vi "WalkThroughExample.vi"() -> ()   [LabVIEW 2019]
uses:
  <vilib>/Rock Robotics/WPI/ThirdParty/JAS_Junk/TrajLib/LINEAR_SYSTEM.ctl
  <vilib>/Analysis/Matrix/Datatypes/RealMatrix.ctl
  <vilib>/Rock Robotics/WPI/ThirdParty/JAS_Junk/TrajLib/DCMOTOR.CTL
  <vilib>/Rock Robotics/WPI/ThirdParty/JAS_Junk/TrajLib/LINEAR_QUADRATIC_REGULATOR.ctl
  <vilib>/Rock Robotics/WPI/ThirdParty/JAS_Junk/TrajLib/KALMAN_FILTER.ctl
  <vilib>/Rock Robotics/WPI/ThirdParty/JAS_Junk/TrajLib/LINEAR_SYSTEM_LOOP.ctl
  <vilib>/Rock Robotics/WPI/ThirdParty/JAS_Junk/TrajLib/LINEAR_PLANT_INV_FF.ctl
  <vilib>/Rock Robotics/WPI/ThirdParty/JAS_Junk/TrajLib/FLYWHEEL_SIM.ctl
  <vilib>/Rock Robotics/WPI/ThirdParty/JAS_Junk/TrajLib/LINEAR_SYSTEM_SIM.ctl
  <vilib>/Rock Robotics/WPI/ThirdParty/JAS_Junk/TrajLib/DCMOTOR_TYPES_ENUM.ctl
  <vilib>/Rock Robotics/WPI/ThirdParty/JAS_Junk/TrajLib/MatBuilder_Create.vi
  <vilib>/Rock Robotics/WPI/ThirdParty/JAS_Junk/TrajLib/DCMotor_GetCIM.vi
  <vilib>/Rock Robotics/WPI/ThirdParty/JAS_Junk/TrajLib/DCMotor_GetAndymark9015.vi
  <vilib>/Rock Robotics/WPI/ThirdParty/JAS_Junk/TrajLib/DCMotor_GetAndymarkRs775_125.vi
  <vilib>/Rock Robotics/WPI/ThirdParty/JAS_Junk/TrajLib/DCMotor_GetBag.vi
  <vilib>/Rock Robotics/WPI/ThirdParty/JAS_Junk/TrajLib/DCMotor_GetBanebotsRs550.vi
  <vilib>/Rock Robotics/WPI/ThirdParty/JAS_Junk/TrajLib/DCMotor_GetBanebotsRs775.vi
  <vilib>/Rock Robotics/WPI/ThirdParty/JAS_Junk/TrajLib/DCMotor_GetFalcon500.vi
  <vilib>/Rock Robotics/WPI/ThirdParty/JAS_Junk/TrajLib/DCMotor_GetMiniCIM.vi
  <vilib>/Rock Robotics/WPI/ThirdParty/JAS_Junk/TrajLib/DCMotor_GetNEO.vi
  <vilib>/Rock Robotics/WPI/ThirdParty/JAS_Junk/TrajLib/DCMotor_GetNEO550.vi
  <vilib>/Rock Robotics/WPI/ThirdParty/JAS_Junk/TrajLib/DCMotor_GetRomiBuiltIn.vi
  <vilib>/Rock Robotics/WPI/ThirdParty/JAS_Junk/TrajLib/DCMotor_GetVex775Pro.vi
  <vilib>/Rock Robotics/WPI/ThirdParty/JAS_Junk/TrajLib/LinearSystem_New.vi
  <vilib>/Rock Robotics/WPI/ThirdParty/JAS_Junk/TrajLib/MatrixHelper_Zero.vi
  <vilib>/Rock Robotics/WPI/ThirdParty/JAS_Junk/TrajLib/MatBuilder_Fill.vi
  <vilib>/Rock Robotics/WPI/ThirdParty/JAS_Junk/TrajLib/Matrix_Ident.vi
  <vilib>/Rock Robotics/WPI/ThirdParty/JAS_Junk/TrajLib/DCMotor_New.vi
  <vilib>/Rock Robotics/WPI/ThirdParty/JAS_Junk/TrajLib/MatrixHelper_CoerceSize.vi
  <vilib>/Analysis/7linalg.llb/Create Special Matrix.vi
  <vilib>/Analysis/7linalg.llb/Create Special Real Matrix.vi
  <vilib>/Rock Robotics/WPI/ThirdParty/JAS_Junk/TrajLib/Trajectory_Library.lvlib
  <vilib>/ptbypt/NI_PtbyPt.lvlib
  <vilib>/Analysis/Matrix/NI_Matrix.lvlib
panel:
  in  "Tab Control":T1(tab)
  out "m_flywheelPlant":T2
  out "Shooter Motor":T4 {"Jr_KgM2" format="%13.5p"; "L_H" format="%13.5p"; "Kt_NMPerAmp" format="%13.5p"; "KvINV_RadPerSecPerVolt" format="%13.5p"; "R_Ohms" format="%13.5p"; "FreeSpeed_RadPerSec" format="%13.5p"; "FreeCurrent_Amps" format="%13.5p"; "StallCurrent_Amps" format="%13.5p"; "StallTorque_NM" format="%13.5p"; "nominalVoltage_Volts" format="%13.5p"}
  out "m_flywheelPlant_ALT":T2
  out "KalmanFilter":T5
  out "Kalman Creation Error":errorcluster
  out "LinearQuadraticRegulator":T6
  out "LQR Creation Error":bool
  out "Linear System Loop":T7
  out "LinSysLoop_Error":bool
  out "Battery Voltage":dbl format="%20.3f"
  out "CO Chart":cluster{dbl, "Voltage":dbl}(graph)
  in  "Shooter \nOn/Off":bool
  out "Encoder Speed\nRad/Sec":dbl(slide) scale=0.0..300.0
  out "Speed \nRad/Sec":dbl format="%16.1f"
  out "Cor Err":bool
  out "Kalman \nFiltered\nSpeed":dbl format="%16.1f"
  out "PV Chart":T9(graph)
  out "Predict Err":bool
  out "Motor Volt \nDmd (CO)":dbl format="%20.3f"
  out "Speed\nSetpoint\nRad/Sec":dbl format="%16.1f"
  out "m_FlyWheelSim":T10 {"GearBox"."Jr_KgM2" format="%13.5p"; "GearBox"."L_H" format="%13.5p"; "GearBox"."Kt_NMPerAmp" format="%13.5p"; "GearBox"."KvINV_RadPerSecPerVolt" format="%13.5p"; "GearBox"."R_Ohms" format="%13.5p"; "GearBox"."FreeSpeed_RadPerSec" format="%13.5p"; "GearBox"."FreeCurrent_Amps" format="%13.5p"; "GearBox"."StallCurrent_Amps" format="%13.5p"; "GearBox"."StallTorque_NM" format="%13.5p"; "GearBox"."nominalVoltage_Volts" format="%13.5p"}
  # "The \"plant\" holds a state-space model of our flywheel. This system has the following properties:\n\n   -  States: [velocity], in radians per second.\n   -  Inputs (what we can \"put in\"): [voltage], in volts.\n   -  Outputs (what we can measure): [velocity], in radians per second.\n\nThere are also constants describing how the system behaves.  For our system these are:\n    Kv ---  Volts per (radian per second)\n    Ka --- Volts per (radian per second squared)\n\n One way the Kv and Ka constants can be found by using the FRC Characterization toolsuite."
  # "<States,States>"
  # "<States,Inputs>"
  # "<Outputs,States>"
  # "<Outputs,Inputs>"
  # "Another way to create a linear system is to use the \"helpers\" available for certain types of systems.\n\nThis uses the following contants:\n   -  DcMotor   --  model cooeficients for a pariticular number of a particular model of motor.\n   -  kFlywheelMomentOfInertia = 0.00032    --    kg * m^2\n   -  kFlywheelGearing = 1.0    --  Reduction between motors and encoder, \n                                     as output over input. If the flywheel spins slower than\n                                     the motors, this number should be greater than one.\n\nThe plant holds a state-space model of our flywheel. This system has the following properties:\n   -  States: [velocity], in radians per second.\n   -  Inputs (what we can \"put in\"): [voltage], in volts.\n   -  Outputs (what we can measure): [velocity], in radians per second."
  # "<States,States>"
  # "<States,Inputs>"
  # "<Outputs,States>"
  # "<Outputs,Inputs>"
  # "Create a Kalman Filter.  This filters the measurment data, by using the \nLinear System model and how accurate we think the model and \nmeasurements are.  \n\nThe parameters are:\n   - States  --  Number of states in the Linear System\n   - Outputs  --  Number of outputs in the Linear System.\n   - State Std Dev  --  How accurate we think our model is\n   - Measurement Std Dev  --  How accurate we think our encoder data is\n   - dtSeconds  --  How often the control loop will be executed."
  # "Steady State Gain  \n<States,Outputs>"
  # "State Estimate <Statess,1>"
  # "<States,States>"
  # "<States,Inputs>"
  # "<Outputs,States>"
  # "<Outputs,Inputs>"
  # "Create the Linear Quadratic Controller.   This takes the measurement input (filtered or not), the desired\nsetpoint (Next R) and calculates the desired motor demand output  U. (Linear System Input) .\n\nCreation of the Linear Quadratic Controller (LQR) takes the following inputs:\n\n   - The Linear System model\n   - Qelms  --  Velocity error tolerance, in radians per second. Decrease\n                         this to more heavily penalize state excursion, or make the controller \n                          behave more aggressively.\n   - Relms  --  Control effort (voltage) tolerance. Decrease this to more\n                        heavily penalize control effort, or make the controller less \n                        aggressive. 12 is a good starting point because that is the \n                        (approximate) maximum voltage of a battery.\n   - dtSeconds  --  Nominal time between loops."
  # "Ref State <States,1>"
  # "Comp and capped \noutput <Inputs,1>"
  # "Controller gain\n<Inputs,States>"
  # "Put everything created so far together into\na Linear System Loop.  This is a convience\nfunction used to help simplify run-time\nexecution."
  # "<States,1>"
  # "<FUTURE --- CLAMP TYPE -- For now\nuse Normalize>"
  # "Steady State Gain  \n<States,Outputs>"
  # "State Estimate <Statess,1>"
  # "<States,States>"
  # "<States,Inputs>"
  # "<Outputs,States>"
  # "<Outputs,Inputs>"
  # "<States,1>"
  # "<Inputs,1>"
  # "<States,Inputs>"
  # "<States,States>"
  # "Ref State <States,1>"
  # "Comp and capped \noutput <Inputs,1>"
  # "Controller gain\n<Inputs,States>"
  # "This code is inside a 20 millisecond loop.\nThe Linear System Loop cluster wire is \nconnected to the left and right side\nof the while loop using a Shift Register\nso the values are continually propagated\nthrough the loop."
  # "The execution steps are:\n\n1) Set the speed setpoint.\n\n2) Feed the current encoder speed measurement to the \n    controller\n\n3) Execute \"Correct\".  In this step the Kalman filter updates \n    the system state vector with the filtered encoder data.\n\n4) Execute \"Predict\".  This updates the LQR controller to \n    generate new voltage commands and use the voltages \n    to predict the next state with out Kalman filter.\n\n5) Get the desirec motor demand.  This is volts.  It will need \n    to be scaled to +/- 1.0 by dividing by 12.0 to send to the \n    motor controller."
  # "This simulates the Flywheel so the encoder speed can\nbe obtained for this example."
  # "<States, 1>"
  # "<Outputs, 1>"
  # "<Inputs, 1>"
  # "<Outputs, 1>"
  # "<States,States>"
  # "<States,Inputs>"
  # "<Outputs,States>"
  # "<Outputs,Inputs>"
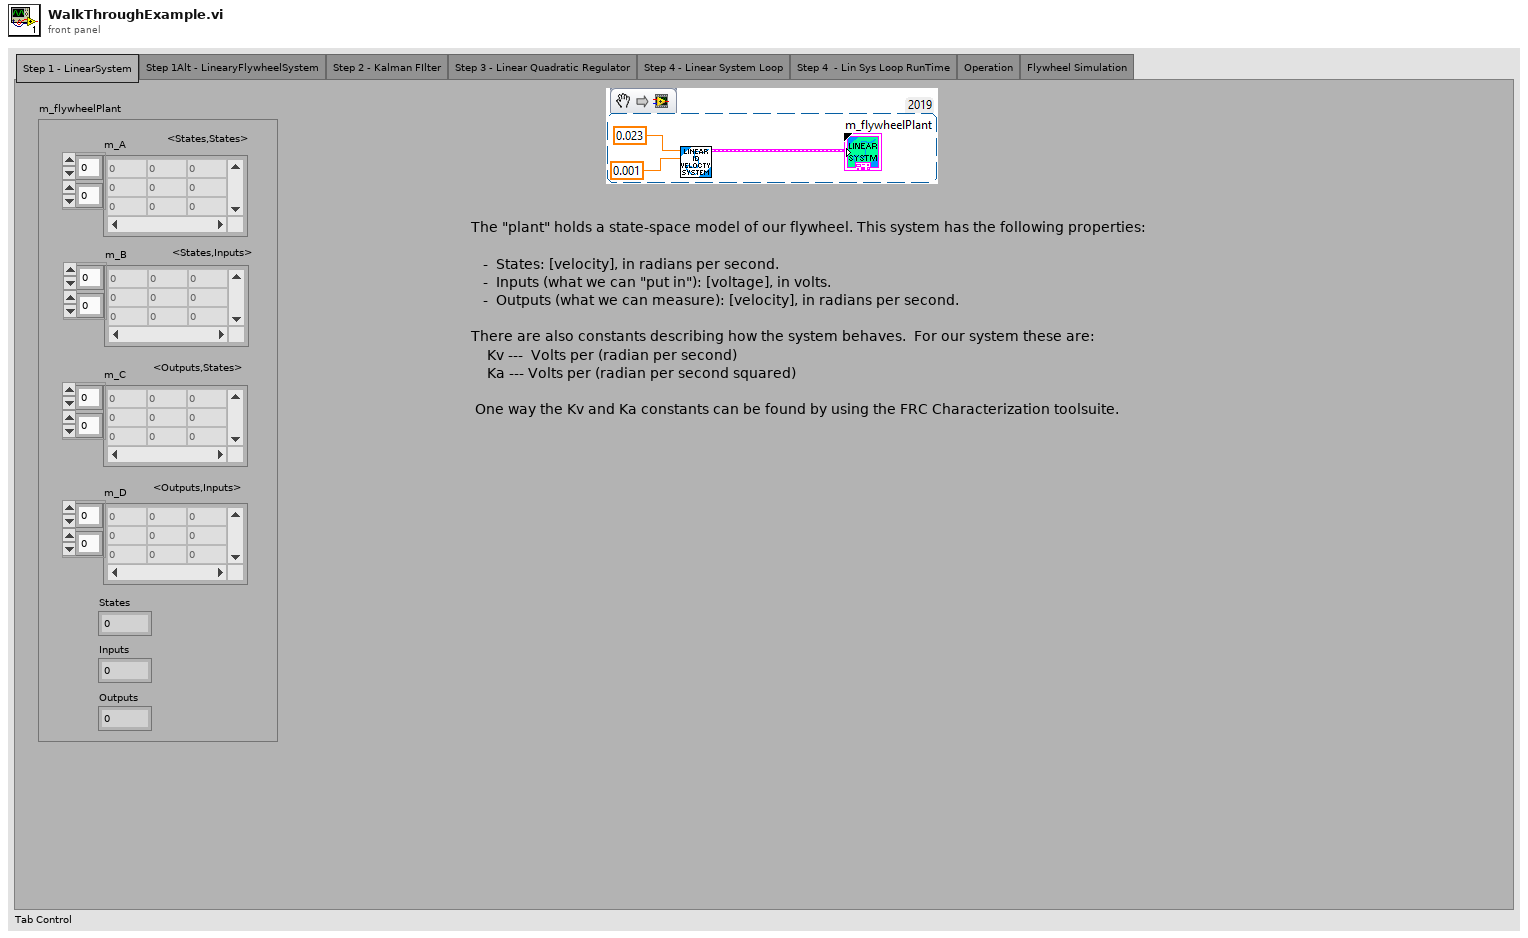
[diagram p1: front panel]
types:
  T1 = enum32{"Step 1 - LinearSystem", "Step 1Alt - LinearyFlywheelSystem", "Step 2 - Kalman FIlter", "Step 3 - Linear Quadratic Regulator", "Step 4 - Linear System Loop", "Step 4  - Lin Sys Loop RunTime", "Operation", "Flywheel Simulation"}
  T2 = typedef "Trajectory_Library.lvlib/LINEAR_SYSTEM.ctl" = cluster{"m_A":T3, "m_B":T3, "m_C":T3, "m_D":T3, "States":i32, "Inputs":i32, "Outputs":i32}
  T3 = typedef "NI_Matrix.lvlib/RealMatrix.ctl" = dbl[][]
  T4 = typedef "Trajectory_Library.lvlib/DCMOTOR.CTL" = cluster{"nominalVoltage_Volts":dbl, "StallTorque_NM":dbl, "StallCurrent_Amps":dbl, "FreeCurrent_Amps":dbl, "FreeSpeed_RadPerSec":dbl, "R_Ohms":dbl, "KvINV_RadPerSecPerVolt":dbl, "Kt_NMPerAmp":dbl, "L_H":dbl, "Jr_KgM2":dbl}
  T5 = typedef "Trajectory_Library.lvlib/KALMAN_FILTER.ctl" = cluster{"m_K":T3, "m_xHat":T3, "States":i32, "Outputs":i32, "m_Plant":T2}
  T6 = typedef "Trajectory_Library.lvlib/LINEAR_QUADRATIC_REGULATOR.ctl" = cluster{"m_r":T3, "m_U":T3, "m_K":T3, "States":i32, "Inputs":i32}
  T7 = typedef "Trajectory_Library.lvlib/LINEAR_SYSTEM_LOOP.ctl" = cluster{"Controller":T6, "FeedForward":T8, "Observer":T5, "Next_R":T3, "Clamp Max":T3}
  T8 = typedef "Trajectory_Library.lvlib/LINEAR_PLANT_INV_FF.ctl" = cluster{"m_R":T3, "m_Uff":T3, "m_B":T3, "m_A":T3, "States":i32, "Inputs":i32}
  T9 = cluster{"upper limit":dbl, "Real Matrix Element":dbl, "Real Matrix Element":dbl}
  T10 = typedef "Trajectory_Library.lvlib/FLYWHEEL_SIM.ctl" = cluster{"LinearSystemSim":T11, "GearBox":T4, "Gearing":dbl}
  T11 = typedef "Trajectory_Library.lvlib/LINEAR_SYSTEM_SIM.ctl" = cluster{"m_Plant":T2, "m_X":T3, "m_Y":T3, "m_U":T3, "MeasureStdDev":T3}
  T12 = typedef "Trajectory_Library.lvlib/DCMOTOR_TYPES_ENUM.ctl" = enum16{"CIM", "AndyMark 9015", "Andy Mark RS 775 125", "Bag", "BaneBots RS 550", "BaneBots RS 775", "Falcon 500", "Mini CIM", "NEO", "NEO 550", "Romi BuiltIn", "Vex 775 Pro"}
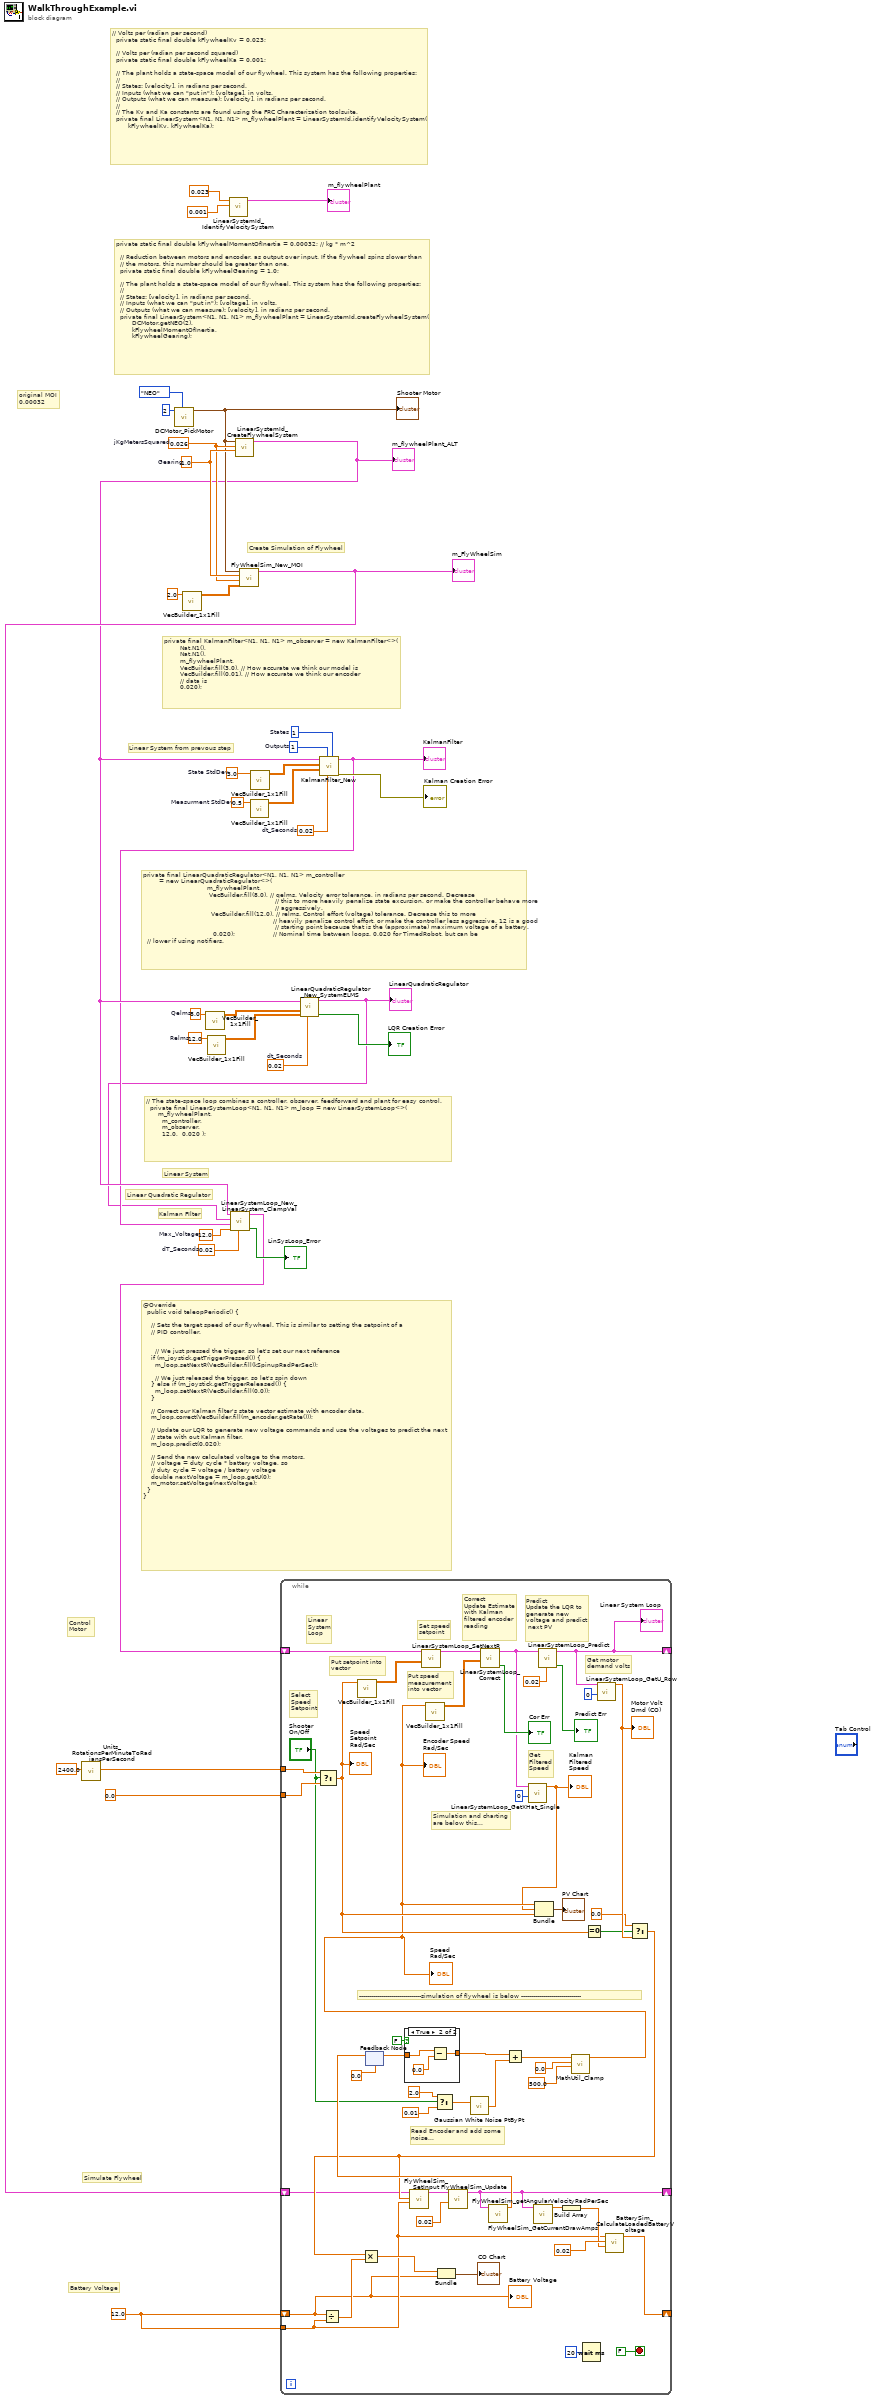
[diagram p0: block diagram]
diagram:
  w10 = 12.0
  w11 = 0.026  # jKgMetersSquared
  w17 = 0.02  # dT_Seconds
  w18 = 12.0  # Max_Voltage
  w22 = 0.02  # dt_Seconds
  w23 = 0.5  # Measurment StdDev
  w24 = 3.0  # State StdDev
  w25 = 1  # States
  w26 = 1  # Outputs
  w30 = 12.0  # Relms
  w31 = 8.0  # Qelms
  w28 = 0.02  # dt_Seconds
  w14 = 1.0  # Gearing
  # "Kalman FIlter"
  # "Linear Quadratic Regulator"
  # "Linear System"
  # "original MOI\n0.00032"
  # "Linear System from prevous step"
  # "Create Simulation of Flywheel"
  # "Control\nMotor"
  # "Simulate Flywheel"
  # "Battery Voltage"
  # "@Override\n  public void teleopPeriodic() {\n\n    // Sets the target speed of our flywheel. This is similar to setting the setpoint of a\n    // PID controller.\n\n\n      // We just pressed the trigger, so let's set our next reference\n    if (m_joystick.getTriggerPressed()) {\n      m_loop.setNextR(VecBuilder.fill(kSpinupRadPerSec));\n\n      // We just released the trigger, so let's spin down\n    } else if (m_joystick.getTriggerReleased()) {\n      m_loop.setNextR(VecBuilder.fill(0.0));\n    }\n\n    // Correct our Kalman filter's state vector estimate with encoder data.\n    m_loop.correct(VecBuilder.fill(m_encoder.getRate()));\n\n    // Update our LQR to generate new voltage commands and use the voltages to predict the next\n    // state with out Kalman filter.\n    m_loop.predict(0.020);\n\n    // Send the new calculated voltage to the motors.\n    // voltage = duty cycle * battery voltage, so\n    // duty cycle = voltage / battery voltage\n    double nextVoltage = m_loop.getU(0);\n    m_motor.setVoltage(nextVoltage);\n  }\n}"
  # "// The state-space loop combines a controller, observer, feedforward and plant for easy control.\n  private final LinearSystemLoop<N1, N1, N1> m_loop = new LinearSystemLoop<>(\n      m_flywheelPlant,\n        m_controller,\n        m_observer,\n        12.0,  0.020 );"
  # "private final LinearQuadraticRegulator<N1, N1, N1> m_controller\n        = new LinearQuadraticRegulator<>(\n                                m_flywheelPlant,\n                                 VecBuilder.fill(8.0), // qelms. Velocity error tolerance, in radians per second. Decrease\n                                                                  // this to more heavily penalize state excursion, or make the controller behave more\n                                                                  // aggressively.\n                                  VecBuilder.fill(12.0), // relms. Control effort (voltage) tolerance. Decrease this to more\n                                                                 // heavily penalize control effort, or make the controller less aggressive. 12 is a good\n                                                                  // starting point because that is the (approximate) maximum voltage of a battery.\n                                   0.020);                   // Nominal time between loops. 0.020 for TimedRobot, but can be\n  // lower if using notifiers."
  # "private final KalmanFilter<N1, N1, N1> m_observer = new KalmanFilter<>(\n        Nat.N1(), \n        Nat.N1(),\n        m_flywheelPlant,\n        VecBuilder.fill(3.0), // How accurate we think our model is\n        VecBuilder.fill(0.01), // How accurate we think our encoder\n        // data is\n        0.020);"
  # "private static final double kFlywheelMomentOfInertia = 0.00032; // kg * m^2\n\n  // Reduction between motors and encoder, as output over input. If the flywheel spins slower than\n  // the motors, this number should be greater than one.\n  private static final double kFlywheelGearing = 1.0;\n\n  // The plant holds a state-space model of our flywheel. This system has the following properties:\n  //\n  // States: [velocity], in radians per second.\n  // Inputs (what we can \"put in\"): [voltage], in volts.\n  // Outputs (what we can measure): [velocity], in radians per second.\n  private final LinearSystem<N1, N1, N1> m_flywheelPlant = LinearSystemId.createFlywheelSystem(\n        DCMotor.getNEO(2),\n        kFlywheelMomentOfInertia,\n        kFlywheelGearing);"
  # "// Volts per (radian per second)\n  private static final double kFlywheelKv = 0.023;\n\n  // Volts per (radian per second squared)\n  private static final double kFlywheelKa = 0.001;\n\n  // The plant holds a state-space model of our flywheel. This system has the following properties:\n  //\n  // States: [velocity], in radians per second.\n  // Inputs (what we can \"put in\"): [voltage], in volts.\n  // Outputs (what we can measure): [velocity], in radians per second.\n  //\n  // The Kv and Ka constants are found using the FRC Characterization toolsuite.\n  private final LinearSystem<N1, N1, N1> m_flywheelPlant = LinearSystemId.identifyVelocitySystem(\n        kFlywheelKv, kFlywheelKa);"
  n1 = call <vilib>:"Units_RotationsPerMinuteToRadiansPerSecond.vi"("RotationsPerMinute"=2400.0) -> ("RadiansPerSecond"=w3:dbl)  [unwired: 10 in]
  n2 = call <vilib>:"DCMotor_PickMotor.vi"("DCMOTOR_TYPES"=DCMOTOR_TYPES_ENUM."NEO", "Num Motors"=2) -> ("DCMOTOR"=w7:T4)  [unwired: 9 in]
  "Shooter Motor" <- w7
  n3 = call <vilib>:"VecBuilder_1x1Fill.vi"("R0_C0"=2.0) -> ("output matrix"=w13:T3)  [unwired: 10 in]
  n4 = call <vilib>:"VecBuilder_1x1Fill.vi"("R0_C0"=w31) -> ("output matrix"=w29:T3)  [unwired: 10 in]
  n5 = call <vilib>:"VecBuilder_1x1Fill.vi"("R0_C0"=w30) -> ("output matrix"=w27:T3)  [unwired: 10 in]
  n6 = call <vilib>:"LinearSystemId_IdentifyVelocitySystem.vi"("kA"=0.001, "kV"=0.023) -> ("Linearsystem"=→"m_flywheelPlant":T2)  [unwired: 8 in, 1 out]
  n7 = call <vilib>:"LinearSystemId_CreateFlywheelSystem.vi"("G"=w14, "jKgMetersSquared"=w11, "DCMOTOR"=w7) -> ("Linearsystem"=w6:T2)  [unwired: 7 in, 1 out]
  "m_flywheelPlant_ALT" <- w6
  n8 = call <vilib>:"FlyWheelSim_New_MOI.vi"("MeasurementStdDev"=w13, "jKgMetersSquared"=w11, "Gearing"=w14, "GearBox"=w7) -> ("FlyWheelSim"=w9:T10)  [unwired: 6 in, 1 out]
  "m_FlyWheelSim" <- w9
  n9 = call <vilib>:"VecBuilder_1x1Fill.vi"("R0_C0"=w23) -> ("output matrix"=w20:T3)  [unwired: 10 in]
  n10 = call <vilib>:"VecBuilder_1x1Fill.vi"("R0_C0"=w24) -> ("output matrix"=w21:T3)  [unwired: 10 in]
  n11 = call <vilib>:"LinearQuadraticRegulator_New_SystemELMS.vi"("dt_Seconds"=w28, "Relms"=w27, "Qelms"=w29, "LINEARSYSTEM"=w6) -> ("Error"=→"LQR Creation Error":bool, "LinearQuadraticRegulator"=w4:T6)  [unwired: 6 in]
  "LinearQuadraticRegulator" <- w4
  n12 = call <vilib>:"KalmanFilter_New.vi"("States"=w25, "dt_Seconds"=w22, "Outputs"=w26, "MeasurementStdDevs"=w20, "StateStdDevs"=w21, "Plant"=w6) -> ("Error"=→"Kalman Creation Error":errorcluster, "KalmanFilter"=w5:T5)  [unwired: 4 in]
  "KalmanFilter" <- w5
  n13 = call <vilib>:"LinearSystemLoop_New_LinearSystem_ClampVal.vi"("dT_Seconds"=w17, "Max_Voltage"=w18, "Observer"=w5, "Controller"=w4, "Plant"=w6) -> ("Error"=→"LinSysLoop_Error":bool, "Linear System Loop"=w1:T7)  [unwired: 5 in]
  n14 = while {
    shift-right: [w37] -> _
    shift-left: w1 -> [w56]
    tunnel: w3 -> [w70]
    tunnel: 0.0 ("R0_C0") -> [w69]
    shift-right: [w66] -> _
    shift-left: w9 -> [w42]
    shift-right: [w61] -> _
    shift-left: w10 -> [w41]
    tunnel: w10 -> [w57]
    stop <- FALSE stop-if-true
    # "Simulation and charting\nare below this..."
    # "Get\nFiltered\nSpeed"
    # "Select\nSpeed\nSetpoint"
    # "Linear\nSystem\nLoop"
    # "-------------------------------simulation of flywheel is below ------------------------------"
    # "Put setpoint into\nvector"
    # "Put speed \nmeasurement\ninto vector"
    # "Set speed\nsetpoint"
    # "Get motor \ndemand volts"
    # "Predict\nUpdate the LQR to \ngenerate new \nvoltage and predict\n next PV"
    # "Correct\nUpdate Estimate\nwith Kalman \nfiltered encoder \nreading"
    # "Read Encoder and add some \nnoise..."
    n15 = Select(t=w70, s="Shooter \nOn/Off", f=w69) -> (s? t:f=w51:dbl)
    "Speed\nSetpoint\nRad/Sec" <- w51
    n16 = Divide(x=w41, y=w57) -> (x/y=w58:dbl)
    n17 = call <vilib>:"VecBuilder_1x1Fill.vi"("R0_C0"=w51) -> ("output matrix"=w55:T3)  [unwired: 10 in]
    n18 = feedback #1(0.0 ("Velocity_RadPerSec")) -> (w68:dbl)
    n19 = case shown="True" FALSE {
      tunnel: w68 -> [w86 w89]
      tunnel: [w86 w88] -> w67
      frame False {
      }
      frame True {
        n20 = Subtract(x=w89, y=0.0) -> (x-y=w88:dbl)
      }
    }
    n21 = call <vilib>:"LinearSystemLoop_SetNextR.vi"("R"=w55, "input inear System Loop"=w56) -> ("out Linear System Loop"=w82:T7)  [unwired: 8 in, 1 out]
    n22 = Select(t=2.0 ("upper bound (100)"), s="Shooter \nOn/Off", f=0.01) -> (s? t:f=w46:dbl)
    n23 = call <vilib>:"Gaussian White Noise PtByPt.vi"("standard deviation"=w46) -> ("Gaussian white noise"=w83:dbl)  [unwired: 2 in]
    n24 = Add(x=w67, y=w83) -> (x+y=w47:dbl)
    n25 = call <vilib>:"MathUtil_Clamp.vi"("High Limit"=500.0, "Low Limit"=0.0, "Value"=w47) -> ("Result"=w40:dbl)  [unwired: 8 in]
    "Encoder Speed\nRad/Sec" <- w40
    "Speed \nRad/Sec" <- w40
    n26 = call <vilib>:"VecBuilder_1x1Fill.vi"("R0_C0"=w40) -> ("output matrix"=w81:T3)  [unwired: 10 in]
    n27 = call <vilib>:"LinearSystemLoop_Correct.vi"("Y"=w81, "input inear System Loop"=w82) -> ("Error"=→"Cor Err":bool, "out Linear System Loop"=w78:T7)  [unwired: 8 in]
    n28 = call <vilib>:"LinearSystemLoop_GetXHat_Single.vi"("Row"=0, "input inear System Loop"=w78) -> ("XHat"=w38:dbl)  [unwired: 9 in]
    "Kalman \nFiltered\nSpeed" <- w38
    n29 = Bundle("Result"=w40, "XHat"=w38, "R0_C0"=w51) -> (→"PV Chart":cluster{"Result":dbl, "XHat":dbl, "R0_C0":dbl})  [unwired: 1 in]
    n30 = call <vilib>:"LinearSystemLoop_Predict.vi"("dT_Seconds"=0.02, "input inear System Loop"=w78) -> ("Error"=→"Predict Err":bool, "out Linear System Loop"=w37:T7)  [unwired: 8 in]
    "Linear System Loop" <- w37
    n31 = Wait (ms)(milliseconds to wait=u32 20) -> ()  [unwired: 1 out]
    n32 = Equal To 0?(x=w51) -> (x = 0?=w52:bool)
    n33 = call <vilib>:"LinearSystemLoop_GetU_Row.vi"("Row"=0, "input inear System Loop"=w37) -> ("U"=w54:dbl)  [unwired: 9 in]
    "Motor Volt \nDmd (CO)" <- w54
    n34 = Select(t=0.0, s=w52, f=w54) -> (s? t:f=w53:dbl)
    n35 = Multiply(x=w53, y=w58) -> (x*y=w60:dbl)
    n36 = call <vilib>:"FlyWheelSim_SetInput.vi"("Battery_Volts"=w57, "Volts"=w53, "FlyWheelSim"=w42) -> ("out FlyWheelSim"=w74:T10)  [unwired: 8 in]
    n37 = Bundle(w60, w41) -> (→"CO Chart":cluster{dbl, dbl})  [unwired: 1 in]
    n38 = call <vilib>:"FlyWheelSim_Update.vi"("dT_Seconds"=0.02, "FlyWheelSim"=w74) -> ("out FlyWheelSim"=w66:T10)  [unwired: 8 in, 1 out]
    n39 = call <vilib>:"FlyWheelSim_getAngularVelocityRadPerSec.vi"("FlyWheelSim"=w66) -> ("Velocity_RadPerSec"=w72:dbl)  [unwired: 10 in]
    n40 = feedback-in #1(w72) -> ()
    n41 = call <vilib>:"FlyWheelSim_GetCurrentDrawAmps.vi"("FlyWheelSim"=w66) -> ("Current_Amps"=w64:dbl)  [unwired: 10 in]
    n42 = Build Array(w64) -> (w63:dbl[])
    n43 = call <vilib>:"BatterySim_CalculateLoadedBatteryVoltage.vi"("Currents"=w63, "Resistance_Ohms"=0.02, "NominalVoltage"=w57) -> ("Voltage"=w61:dbl)  [unwired: 8 in]
    "Battery Voltage" <- w41
  }
